vi "Post-Process.vi"(11 "Element in":refnum<class "Element.lvclass">) -> (2 "New Elements":refnum<class "Element.lvclass">[](array[class]), 3 "Element out":refnum<class "Element.lvclass">)   [LabVIEW 2021, in "Element.lvclass"]
uses:
  Element.lvclass
  Element.lvclass/Element.ctl
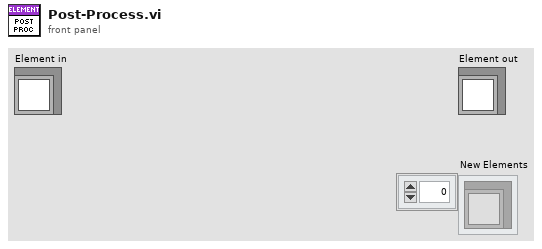
[diagram p1: front panel]
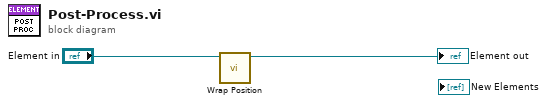
[diagram p0: block diagram]
diagram:
  n1 = call "Wrap Position.vi"("Movable in"="Element in") -> ("Movable out"=→"Element out":refnum<class "Element.lvclass">)  [unwired: 10 in]
